vi "Pre Launch Init.vi"(11 "Nested in":refnum<class "MSS Remote Actor.lvclass">) -> (0 "error out":errorcluster, 3 "Nested out":refnum<class "MSS Remote Actor.lvclass">)   [LabVIEW 2023, in "MSS Remote Actor.lvlib" / "MSS Remote Actor.lvclass"]
doc: "(<B>Filename</B>: Actor Framework.lvlib:Actor.lvclass:Pre Launch Init.vi)\n\nDefines behavior that occurs after the Launch Nested Actor method is invoked but before the actor's Actor Core method begins running.\n\nBy default, this method does nothing. A descendant class may override it to define behavior."
uses:
  MSS Remote Actor.lvclass
  MSS Remote Actor.lvclass/MSS Remote Actor.ctl
  Actor-Layers/Actor Log Error to Harddrive/Actor Log Error to Harddrive.lvclass
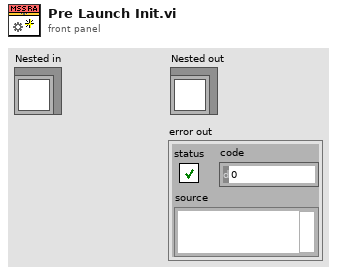
[diagram p1: front panel]
types:
  T1 = cluster{"Phys Instr CFGs":string[], "Virt Instrs CFG":string}
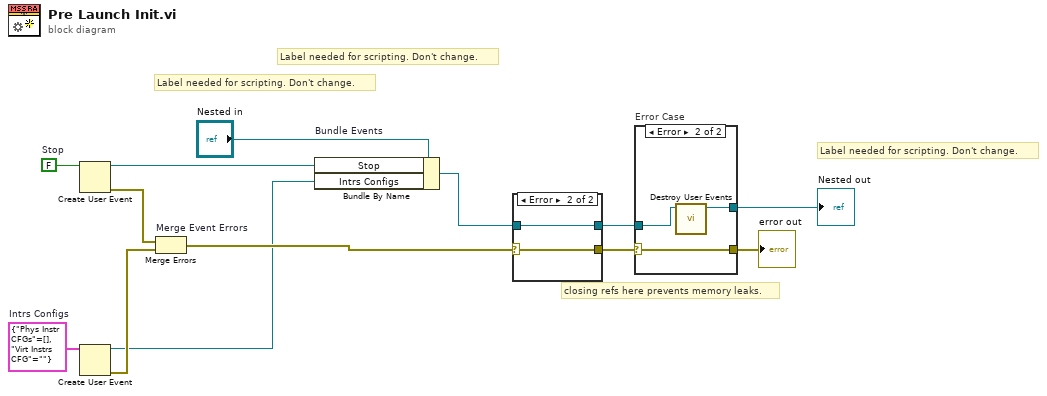
[diagram p0: block diagram]
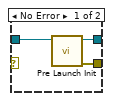
[diagram p2: hidden frame]
diagram:
  w2 = T1 {"Phys Instr CFGs"=[], "Virt Instrs CFG"=""}  # Intrs Configs
  w12 = FALSE  # Stop
  # "Label needed for scripting. Don't change."
  # "Label needed for scripting. Don't change."
  # "Label needed for scripting. Don't change."
  # "closing refs here prevents memory leaks."
  n1 = Create User Event(user event datatype=w12) -> (user event=w9:refnum<user-event>, error out=w11:errorcluster)  [unwired: 1 in]
  n2 = Create User Event(user event datatype=w2) -> (user event=w1:refnum<user-event>, error out=w5:errorcluster)  [unwired: 1 in]
  n3 = Merge Errors "Merge Event Errors"(w11, w5) -> (w4:errorcluster)
  n4 = Bundle By Name "Bundle Events"(cluster="Nested in", "Stop"=w9, "Intrs Configs"=w1) -> (w3:refnum<class "MSS Remote Actor.lvclass">)
  n5 = case shown="Error" w4 {
    selector: w4 -> [_ w18]
    tunnel: [w16 w17] -> w7
    tunnel: [w15 w18] -> w6
    tunnel: w3 -> [w14 w17]
    frame No Error {
      n6 = call-parent "Pre Launch Init.vi"("Actor in"=w14) -> ("error out"=w15:errorcluster, "Actor out"=w16:refnum<class "MSS Remote Actor.lvclass">)  [unwired: 9 in]
    }
    frame Error {
    }
  }
  n7 = case "Error Case" shown="Error" w6 {
    selector: w6 -> [w19 w23]
    tunnel: w7 -> [w20 w22]
    tunnel: [w20 w21] -> w10
    tunnel: [w19 w23] -> w8
    frame No Error {
    }
    frame Error {
      n8 = call "Destroy User Events.vi"("UI Template in"=w22) -> ("UI Template out"=w21:refnum<class "MSS Remote Actor.lvclass">)  [unwired: 10 in]
    }
  }
  "error out" <- w8
  "Nested out" <- w10
